vi "Save test data.vi"(8 "error in":errorcluster, 9 "Parttype":T1, 10 "SN":string, 11 "ECU Info":T2) -> (0 "error out":errorcluster)   [LabVIEW 2014]
uses:
  typedefs/parttype.ctl
  <vilib>/Utility/file.llb/Write To Spreadsheet File (string).vi
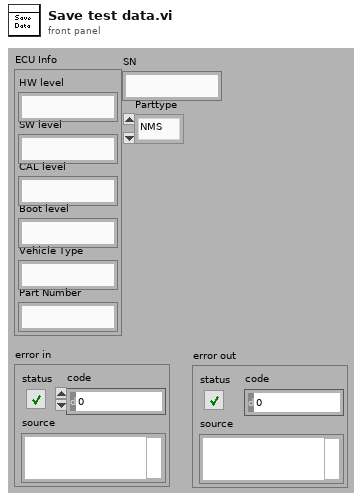
[diagram p1: front panel]
types:
  T1 = typedef "parttype.ctl" = enum16{"NMS", "B-SUV"}
  T2 = cluster{"HW level":string, "SW level":string, "CAL level":string, "Boot level":string, "Vehicle Type":string, "Part Number":string}
  T3 = cluster{"ECU Info":cluster{"HW level":string, "SW level":string, "CAL level":string, "Boot level":string, "Vehicle Type":string, "Part Number":string}, "Manual Print":bool, "SN":string}
  T4 = cluster{"Base Path":path, "Excel Data Array":string[], "ECU Info":cluster{"HW level":string, "SW level":string, "CAL level":string, "Boot level":string, "Vehicle Type":string, "Part Number":string}, "SN":string, "Parttype":T1, "Date n Time":string}
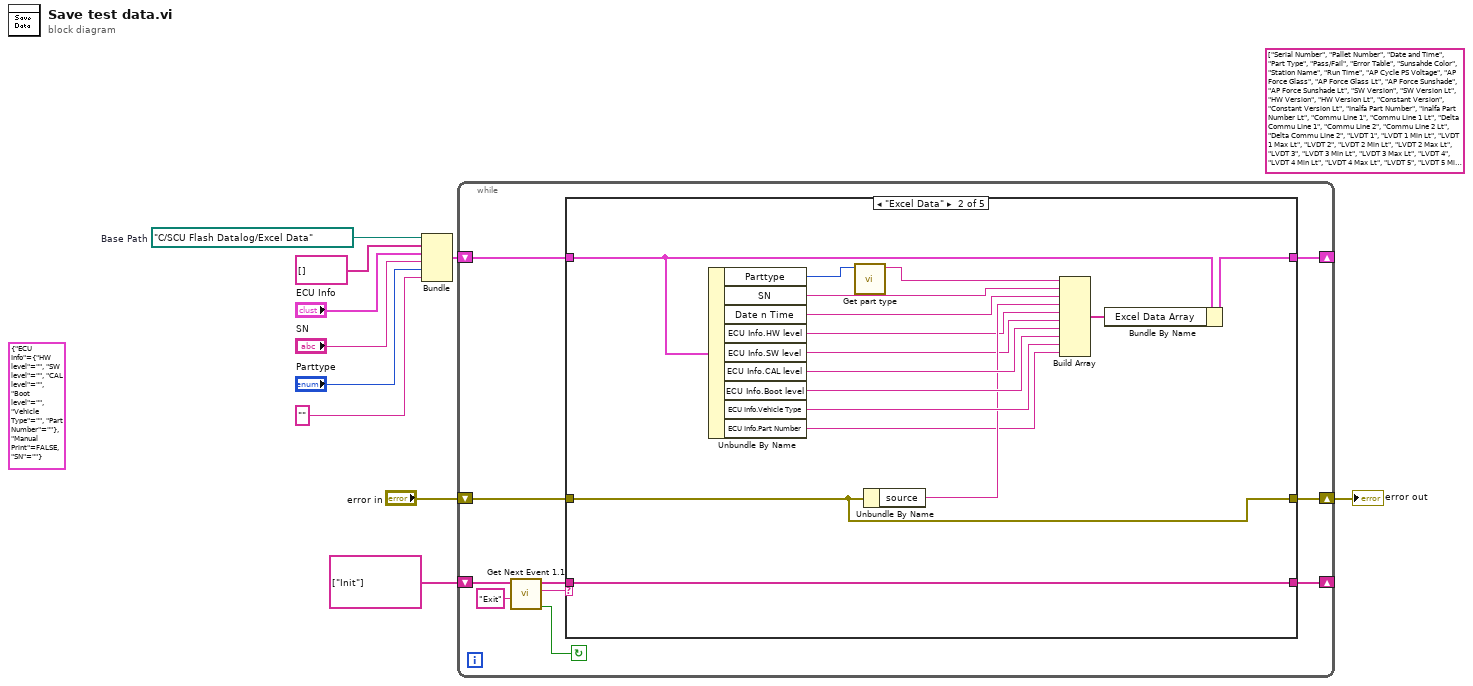
[diagram p0: block diagram]
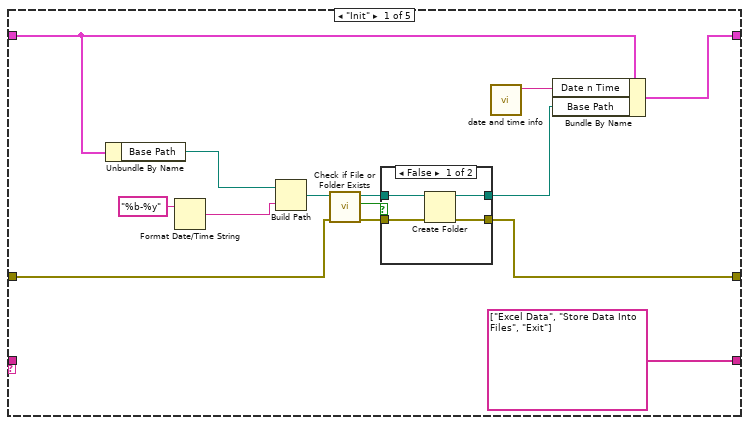
[diagram p2: hidden frame]
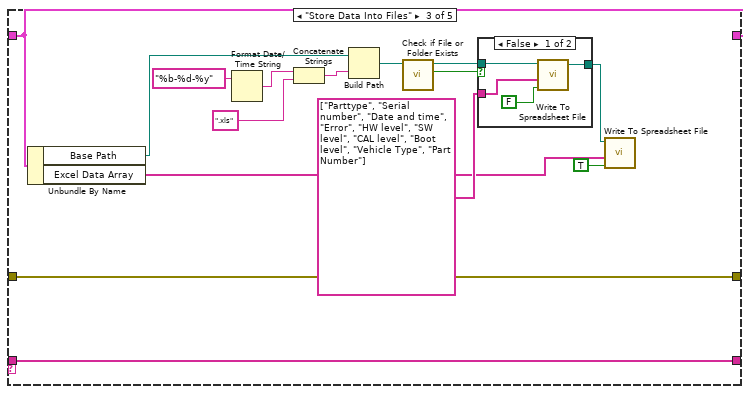
[diagram p4: hidden frame]
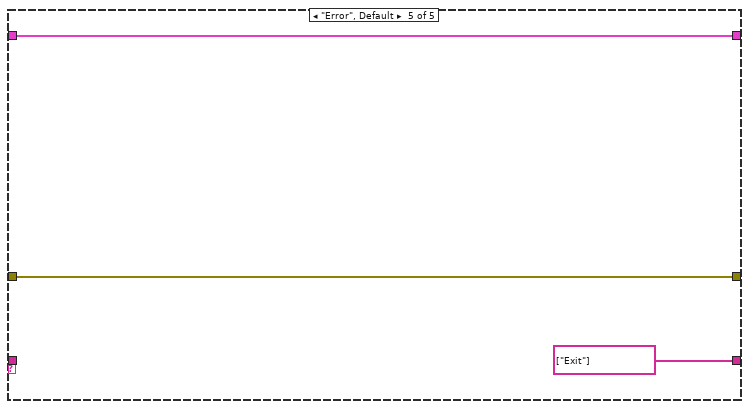
[diagram p7: hidden frame]
diagram:
  (unwired) T3 {"ECU Info"={"HW level"="", "SW level"="", "CAL level"="", "Boot level"="", "Vehicle Type"="", "Part Number"=""}, "Manual Print"=FALSE, "SN"=""}
  (unwired) string[] ["Serial Number", "Pallet Number", "Date and Time", "Part Type", "Pass/Fail", "Error Table", "Sunsahde Color", "Station Name", "Run Time", "AP Cycle PS Voltage", "AP Force Glass", "AP Force Glass Lt", "AP Force Sunshade", "AP Force Sunshade Lt", "SW Version", "SW Version Lt", "HW Version", "HW Version Lt", "Constant Version", "Constant Version Lt", "Inalfa Part Number", "Inalfa Part Number Lt", "Commu Line 1", "Commu Line 1 Lt", "Delta Commu Line 1", "Commu Line 2", "Commu Line 2 Lt", "Delta Commu Line 2", "LVDT 1", "LVDT 1 Min Lt", "LVDT 1 Max Lt", "LVDT 2", "LVDT 2 Min Lt", "LVDT 2 Max Lt", "LVDT 3", "LVDT 3 Min Lt", "LVDT 3 Max Lt", "LVDT 4", "LVDT 4 Min Lt", "LVDT 4 Max Lt", "LVDT 5", "LVDT 5 Min Lt", "LVDT 5 Max Lt", "LVDT 6", "LVDT 6 Min Lt", "LVDT 6 Max Lt", "LVDT 7", "LVDT 7 Min Lt", "LVDT 7 Max Lt", "LVDT 8", "LVDT 8 Min Lt", "LVDT 8 Max Lt", "LVDT 9", "LVDT 9 Min Lt", "LVDT 9 Max Lt", "LVDT 10", "LVDT 10 Min Lt", "LVDT 10 Max Lt", "LVDT 11", "LVDT 11 Min Lt", "LVDT 11 Max Lt", "LVDT 12", "LVDT 12 Min Lt", "LVDT 12 Max Lt", "LVDT 13", "LVDT 13 Min Lt", "LVDT 13 Max Lt", "LVDT 14", "LVDT 14 Min Lt", "LVDT 14 Max Lt", "iGPS LVDT 1", "iGPS LVDT 1 Min Lt", "iGPS LVDT 1 Max Lt", "iGPS LVDT 2", "iGPS LVDT 2 Min Lt", "iGPS LVDT 2 Max Lt", "iGPS LVDT 3", "iGPS LVDT 3 Min Lt", "iGPS LVDT 3 Max Lt", "iGPS LVDT 4", "iGPS LVDT 4 Min Lt", "iGPS LVDT 4 Max Lt", "iGPS LVDT 5", "iGPS LVDT 5 Min Lt", "iGPS LVDT 5 Max Lt", "iGPS LVDT 6", "iGPS LVDT 6 Min Lt", "iGPS LVDT 6 Max Lt", "iGPS LVDT 7", "iGPS LVDT 7 Min Lt", "iGPS LVDT 7 Max Lt", "iGPS LVDT 8", "iGPS LVDT 8 Min Lt", "iGPS LVDT 8 Max Lt", "iGPS LVDT 9", "iGPS LVDT 9 Min Lt", "iGPS LVDT 9 Max Lt", "iGPS LVDT 10", "iGPS LVDT 10 Min Lt", "iGPS LVDT 10 Max Lt", "iGPS LVDT 11", "iGPS LVDT 11 Min Lt", "iGPS LVDT 11 Max Lt", "iGPS LVDT 12", "iGPS LVDT 12 Min Lt", "iGPS LVDT 12 Max Lt", "iGPS LVDT 13", "iGPS LVDT 13 Min Lt", "iGPS LVDT 13 Max Lt", "iGPS LVDT 14", "iGPS LVDT 14 Min Lt", "iGPS LVDT 14 Max Lt", "SH Close Min", "SH Close Min Lt", "SH Close Max", "SH Close Max Lt", "SH Close Avg Min", "SH Close Avg Min Lt", "SH Close Avg Max", "SH Close Avg Max Lt", "SH Close Variance", "SH Close Variance Lt", "SH Close Noise Check?", "SH Open Min", "SH Open Min Lt", "SH Open Max", "SH Open Max Lt", "SH Open Avg Min", "SH Open Avg Min Lt", "SH Open Avg Max", "SH Open Avg Max Lt", "SH Open Variance", "SH Open Variance Lt", "SH Open Noise Check?", "AP Vent Force", "AP Vent Force Min Lt", "AP Vent Force Max Lt", "Spare Field 1", "Spare Field 2", "Spare Field 3", "Spare Field 4", "Spare Field 5", "Spare Field 6", "Spare Field 7", "Motion", "PS Voltage", "Switch 1", "Switch 2", "Switch 3", "Switch 4", "Switch 5", "Switch 6", "Switch 7", "Switch 8", "Avg Current", "Avg Current Min Lt", "Avg Current Max Lt", "Run Time", "Run Time Max", "Speed", "Speed Min Lt", "Noise Test Tested?", "Motion", "PS Voltage", "Switch 1", "Switch 2", "Switch 3", "Switch 4", "Switch 5", "Switch 6", "Switch 7", "Switch 8", "Avg Current", "Avg Current Min Lt", "Avg Current Max Lt", "Run Time", "Run Time Max", "Speed", "Speed Min Lt", "Noise Test Tested?", "Motion", "PS Voltage", "Switch 1", "Switch 2", "Switch 3", "Switch 4", "Switch 5", "Switch 6", "Switch 7", "Switch 8", "Avg Current", "Avg Current Min Lt", "Avg Current Max Lt", "Run Time", "Run Time Max", "Speed", "Speed Min Lt", "Noise Test Tested?", "Motion", "PS Voltage", "Switch 1", "Switch 2", "Switch 3", "Switch 4", "Switch 5", "Switch 6", "Switch 7", "Switch 8", "Avg Current", "Avg Current Min Lt", "Avg Current Max Lt", "Run Time", "Run Time Max", "Speed", "Speed Min Lt", "Noise Test Tested?", "Motion", "PS Voltage", "Switch 1", "Switch 2", "Switch 3", "Switch 4", "Switch 5", "Switch 6", "Switch 7", "Switch 8", "Avg Current", "Avg Current Min Lt", "Avg Current Max Lt", "Run Time", "Run Time Max", "Speed", "Speed Min Lt", "Noise Test Tested?", "Motion", "PS Voltage", "Switch 1", "Switch 2", "Switch 3", "Switch 4", "Switch 5", "Switch 6", "Switch 7", "Switch 8", "Avg Current", "Avg Current Min Lt", "Avg Current Max Lt", "Run Time", "Run Time Max", "Speed", "Speed Min Lt", "Noise Test Tested?", "Motion", "PS Voltage", "Switch 1", "Switch 2", "Switch 3", "Switch 4", "Switch 5", "Switch 6", "Switch 7", "Switch 8", "Avg Current", "Avg Current Min Lt", "Avg Current Max Lt", "Run Time", "Run Time Max", "Speed", "Speed Min Lt", "Noise Test Tested?", "Motion", "PS Voltage", "Switch 1", "Switch 2", "Switch 3", "Switch 4", "Switch 5", "Switch 6", "Switch 7", "Switch 8", "Avg Current", "Avg Current Min Lt", "Avg Current Max Lt", "Run Time", "Run Time Max", "Speed", "Speed Min Lt", "Noise Test Tested?", "Motion", "PS Voltage", "Switch 1", "Switch 2", "Switch 3", "Switch 4", "Switch 5", "Switch 6", "Switch 7", "Switch 8", "Avg Current", "Avg Current Min Lt", "Avg Current Max Lt", "Run Time", "Run Time Max", "Speed", "Speed Min Lt", "Noise Test Tested?", "Motion", "PS Voltage", "Switch 1", "Switch 2", "Switch 3", "Switch 4", "Switch 5", "Switch 6", "Switch 7", "Switch 8", "Avg Current", "Avg Current Min Lt", "Avg Current Max Lt", "Run Time", "Run Time Max", "Speed", "Speed Min Lt", "Noise Test Tested?"] ("all rows")
  w9 = path "C:/SCU Flash Datalog/Excel Data"  # Base Path
  n1 = Bundle("Base Path"=w9, "Excel Data Array"=string[] [], "ECU Info"="ECU Info", "SN"="SN", "Parttype"="Parttype", "Date n Time"="") -> (w6:T4)  [unwired: 1 in]
  n2 = while {
    shift-right: [w17] -> _
    shift-left: string[] ["Init"] ("event queue out") -> [w16]
    shift-right: [w14] -> _
    shift-left: w6 -> [w15]
    shift-right: [w11] -> w7
    shift-left: "error in" -> [w12]
    stop <- w20 continue-if-true
    n3 = call "Get Next Event 1.1.vi"("Exit Event"="Exit", "event queue in"=w16) -> ("Condition (Exit:F)"=w20:bool, "next event"=w19:string, "event queue out"=w18:string[])  [unwired: 6 in, 1 out]
    n4 = case shown="\"Excel Data\"" w19 {
      tunnel: w18 -> [_ w56 w70 w78 _]
      tunnel: [string[] ["Excel Data", "Store Data Into Files", "Exit"] ("event queue out") w56 w70 w78 string[] ["Exit"] ("event queue out")] -> w17
      tunnel: w15 -> [w29 w54 w59 w79 w82]
      tunnel: [w34 w53 w59 w79 w82] -> w14
      tunnel: w12 -> [w24 w41 w57 w77 w80]
      tunnel: [w23 w41 w57 w77 w80] -> w11
      frame "Init" {
        n5 = Unbundle By Name(w29) -> ("Base Path"=w28:path)
        n6 = Format Date/Time String(time format string (%c)="%b-%y") -> (date/time string=w21:string)  [unwired: 2 in]
        n7 = Build Path(base path=w28, name or relative path=w21) -> (appended path=w30:path)
        n8 = call <vilib>:"Check if File or Folder Exists.vi"("error in (no error)"=w24, "path"=w30) -> ("error out"=w25:errorcluster, "file or folder exists?"=w27:bool, "dup path"=w26:path)  [unwired: 7 in]
        n9 = case shown="False" w27 {
          tunnel: w26 -> [w38 w39]
          tunnel: w25 -> [w37 w40]
          tunnel: [w36 w40] -> w23
          tunnel: [w35 w39] -> w22
          frame False {
            n10 = Create Folder(path (use dialog)=w38, error in=w37) -> (created path=w35:path, error out=w36:errorcluster)  [unwired: 1 in, 1 out]
          }
          frame True {
          }
        }
        n11 = call "date and time info.vi"() -> ("Output String"=w32:string)  [unwired: 11 in]
        n12 = Bundle By Name(cluster=w29, "Date n Time"=w32, "Base Path"=w22) -> (w34:T4)
      }
      frame "Excel Data" {
        n13 = Unbundle By Name(w54) -> ("Parttype"=w48:T1, "SN"=w55:string, "Date n Time"=w51:string, "ECU Info.HW level"=w45:string, "ECU Info.SW level"=w44:string, "ECU Info.CAL level"=w52:string, "ECU Info.Boot level"=w49:string, "ECU Info.Vehicle Type"=w50:string, "ECU Info.Part Number"=w43:string)
        n14 = call "Get part type.vi"("Enum"=w48) -> ("Parttype"=w47:string)  [unwired: 10 in]
        n15 = Unbundle By Name(w41) -> ("source"=w46:string)
        n16 = Build Array(w47, w55, w51, w46, w45, w44, w52, w49, w50, w43) -> (w42:string[])
        n17 = Bundle By Name(cluster=w54, "Excel Data Array"=w42) -> (w53:T4)
      }
      frame "Store Data Into Files" {
        n18 = Unbundle By Name(w59) -> ("Base Path"=w58:path, "Excel Data Array"=w61:string[])
        n19 = Format Date/Time String(time format string (%c)="%b-%d-%y") -> (date/time string=w68:string)  [unwired: 2 in]
        n20 = Concatenate Strings(w68, ".xls" ("string")) -> (w63:string)
        n21 = Build Path(base path=w58, name or relative path=w63) -> (appended path=w66:path)
        n22 = call <vilib>:"Check if File or Folder Exists.vi"("path"=w66) -> ("file or folder exists?"=w65:bool, "dup path"=w64:path)  [unwired: 8 in, 1 out]
        n23 = case shown="False" w65 {
          tunnel: w64 -> [w75 w76]
          tunnel: [w74 w76] -> w60
          tunnel: string[] ["Parttype", "Serial number", "Date and time", "Error", "HW level", "SW level", "CAL level", "Boot level", "Vehicle Type", "Part Number"] ("all rows") -> [w73 _]
          frame False {
            n24 = call-poly <vilib>:"Write To Spreadsheet File.vi"("append to file? (new file:F)"=FALSE, "1D data"=w73, "file path (dialog if empty)"=w75) -> ("new file path (Not A Path if cancelled)"=w74:path)  [unwired: 5 in]
          }
          frame True {
          }
        }
        n25 = call-poly <vilib>:"Write To Spreadsheet File.vi"("append to file? (new file:F)"=TRUE, "1D data"=w61, "file path (dialog if empty)"=w60) -> ()  [unwired: 5 in, 1 out]
      }
      frame "Exit" {
      }
      frame "Error", Default {
      }
    }
  }
  "error out" <- w7
